vi "ExampleVI_GetSetParameter.vi"() -> ()   [LabVIEW 2013]
panel:
  out "Atmpshere Correction":bool
  out "Humidity":sgl
  in  "HUMIDITY":sgl=30.0
  in  "ATMOSPHERECORRECTION":bool
  in  "GETPARAMETER - Button":bool
  out "Boolesch":bool
  in  "EXIT - Button":bool
  in  "Menüring":u32(ring) items=["t885-1(2078204)"=2078204]
  in  "CONNECT - BUTTON":bool
  out "Fehler (Ausgang)":errorcluster caption="ErrorOut"
  # "SET PARAMETER"
  # "Humidity"
  # "Atmosphere Correction"
  # "Humidity"
  # "Atmosphere Correction"
  # "CONNECTION"
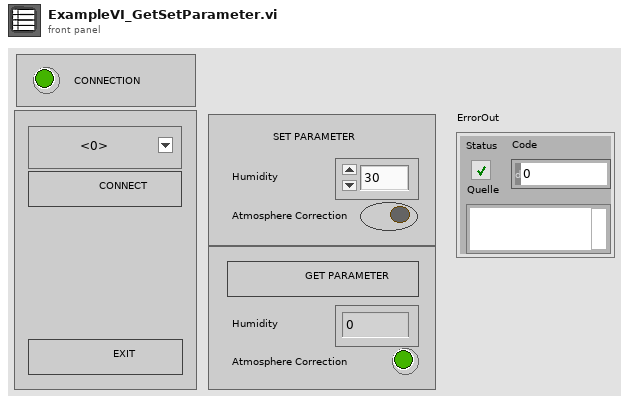
[diagram p1: front panel]
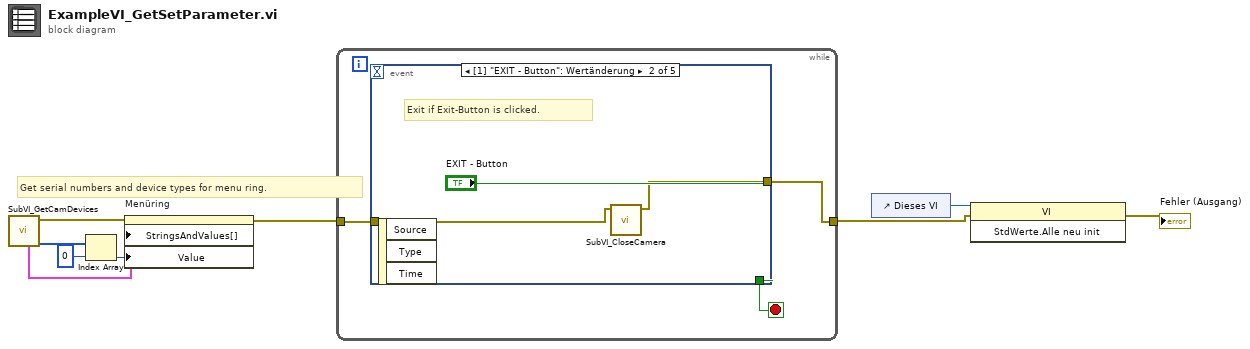
[diagram p0: block diagram]
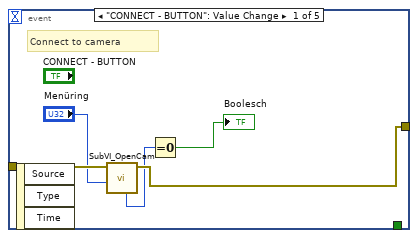
[diagram p2: hidden frame]
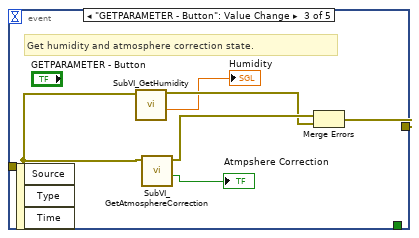
[diagram p3: hidden frame]
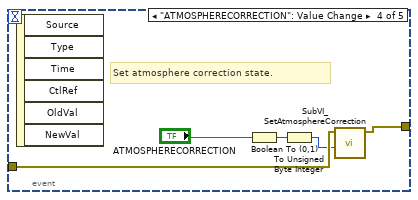
[diagram p4: hidden frame]
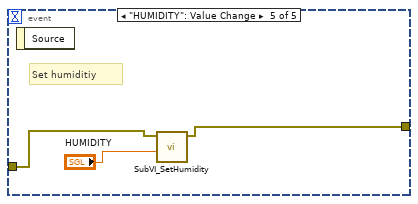
[diagram p5: hidden frame]
diagram:
  # "Get serial numbers and device types for menu ring."
  n1 = call "SubVI_GetCamDevices.vi"() -> ("au32CameraSerials"=w6:u32[], "ErrorOut"=w8:errorcluster, "strCameraDeviceType"=w4:cluster{string, "Output":u32}[])  [unwired: 7 in, 2 out]
  n2 = Index Array(array=w6, index=0 ("Index")) -> (element=w5:u32)
  n3 = property on="Menüring" class="Ring (strikt)"(error in=w8, "StringsAndValues[]"=w4, "Value"=w5) -> (error out=w9:errorcluster)  [unwired: 1 in, 1 out]
  n4 = while {
    tunnel: w9 -> [w12]
    tunnel: [w10] -> w2
    stop <- w11 stop-if-true
    n5 = event shown="[1] \"EXIT - Button\": Wertänderung" {
      selector: _ -> [_ _ _ _ _]
      dyn-events: _ -> [_ _ _ _ _]
      timeout: _ -> [_ _ _ _ _]
      tunnel: w12 -> [w15 w19 w26 w28 w34]
      tunnel: [w16 w18 w23 w29 w33] -> w10
      tunnel: [_ "EXIT - Button" _ _ _] -> w11
      event "CONNECT - BUTTON": Value Change {
        # "Connect to camera"
        n6 = event-data() -> ()  [unwired: 1 in, 3 out]
        n7 = call "SubVI_OpenCam.vi"("u32SerialNumber"="Menüring", "ErrorIn"=w15) -> ("ErrorOut"=w16:errorcluster, "u8Status"=w13:u8)  [unwired: 8 in]
        n8 = Equal To 0?(x=w13) -> (x = 0?=→"Boolesch":bool)
      }
      event "EXIT - Button": Value Change {
        # "Exit if Exit-Button is clicked."
        n9 = event-data() -> ()  [unwired: 1 in, 3 out]
        n10 = call "SubVI_CloseCamera.vi"("ErrorIn"=w19) -> ("ErrorOut"=w18:errorcluster)  [unwired: 9 in, 1 out]
      }
      event "GETPARAMETER - Button": Value Change {
        # "Get humidity and atmosphere correction state."
        n11 = event-data() -> ()  [unwired: 1 in, 3 out]
        n12 = call "SubVI_GetHumidity.vi"("ErrorIn"=w26) -> ("fHumidity"=→"Humidity":sgl, "ErrorOut"=w24:errorcluster)  [unwired: 8 in, 1 out]
        n13 = call "SubVI_GetAtmosphereCorrection.vi"("ErrorIn"=w26) -> ("bAtmosCorrEnable"=→"Atmpshere Correction":bool, "ErrorOut"=w25:errorcluster)  [unwired: 8 in, 1 out]
        n14 = Merge Errors(w25, w24) -> (w23:errorcluster)
      }
      event "ATMOSPHERECORRECTION": Value Change {
        # "Set atmosphere correction state."
        n15 = event-data() -> ()  [unwired: 1 in, 6 out]
        n16 = Boolean To (0,1)(Boolean="ATMOSPHERECORRECTION") -> (0, 1=w30:i16)
        n17 = To Unsigned Byte Integer(number=w30) -> (unsigned 8bit integer=w27:u8)
        n18 = call "SubVI_SetAtmosphereCorrection.vi"("u8AtmosCorrEnable"=w27, "ErrorIn"=w28) -> ("ErrorOut"=w29:errorcluster)  [unwired: 8 in, 1 out]
      }
      event "HUMIDITY": Value Change {
        # "Set humiditiy"
        n19 = event-data() -> ()  [unwired: 1 in, 1 out]
        n20 = call "SubVI_SetHumidity.vi"("fHumidity"="HUMIDITY", "ErrorIn"=w34) -> ("ErrorOut"=w33:errorcluster)  [unwired: 8 in, 1 out]
      }
    }
  }
  n21 = control-ref of="Dieses VI"() -> (w3:refnum<vi>)
  n22 = invoke class="VI" method="StdWerte.Alle neu init"(reference=w3, error in=w2) -> (error out=→"Fehler (Ausgang)":errorcluster)  [unwired: 1 in, 2 out]
